vi "tirf-initialize-handle.vi"() -> (3 "handle":i32)   [LabVIEW 2014]
uses:
  Library Files - Andor and MadCity/TIRF/TIRF-Lock.dll
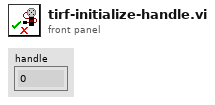
[diagram p1: front panel]
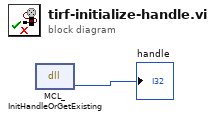
[diagram p0: block diagram]
diagram:
  n1 = dll-call lib="C:/Users/Lambda2/Desktop/Testing/Testing-Lambda/TIRF-Microscope/Library Files - Andor and MadCity/TIRF/TIRF-Lock.dll" fn="MCL_InitHandleOrGetExisting"() -> ("handle"=→"handle":i32)  [unwired: 3 in, 2 out]
